vi "TDT-Status.vi"(0 "Data":T1={"TTankX"=refnum, "TDevAccX"=refnum, "LastTime"=0.0, "error"={"status"=FALSE, "code"=0, "source"=""}, "Block Name"="", "Circuit Tag"="", "Tank Name"="", "NumTicks"=0, "LastTick"=0.0, "Idle?"=FALSE, "Wait (ms)"=1000, "LastArtf"=0.0, "LastTosc"=0.0}, 11 "error in (no error)":errorcluster) -> (8 "SysMode":i32, 15 "error out":errorcluster)   [LabVIEW 2015]
uses:
  TDT Interface Data.ctl
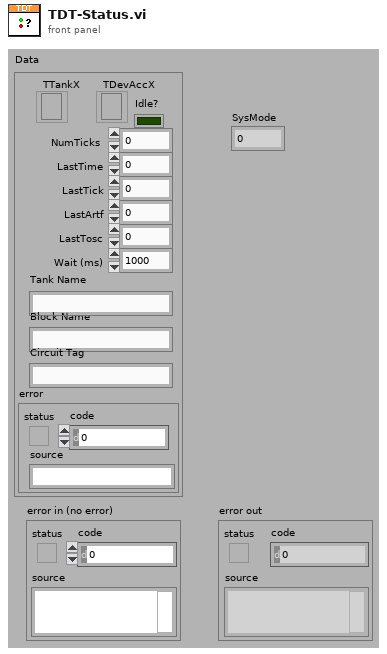
[diagram p1: front panel]
types:
  T1 = typedef "TDT Interface Data.ctl" = cluster{"TTankX":refnum<k7>, "TDevAccX":refnum<k7>, "LastTime":dbl, "error":errorcluster, "Block Name":string, "Circuit Tag":string, "Tank Name":string, "NumTicks":i32, "LastTick":dbl, "Idle?":bool, "Wait (ms)":u32, "LastArtf":dbl, "LastTosc":dbl}
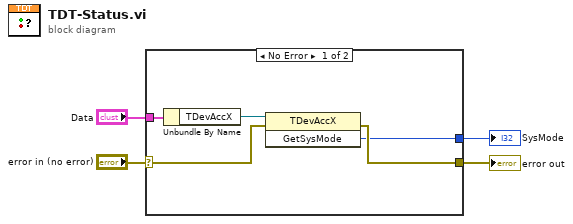
[diagram p0: block diagram]
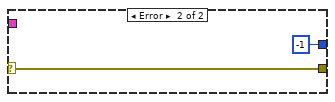
[diagram p2: hidden frame]
diagram:
  n1 = case shown="No Error" "error in (no error)" {
    selector: "error in (no error)" -> [w7 w11]
    tunnel: [w6 w11] -> w3
    tunnel: "Data" -> [w9 _]
    tunnel: [w5 -1 ("GetSysMode")] -> w1
    frame No Error {
      n2 = Unbundle By Name(w9) -> ("TDevAccX"=w8:refnum<k7>)
      n3 = invoke class="TDevAccX" method="GetSysMode"(reference=w8, error in=w7) -> (error out=w6:errorcluster, "GetSysMode"=w5:i32)  [unwired: 1 in, 1 out]
    }
    frame Error {
    }
  }
  "error out" <- w3
  "SysMode" <- w1
